vi "시뮬레이터_0720.vi"() -> ()   [LabVIEW 2017]
doc: "This example demonstrates how to continuously acquire buffered voltage measurements using a DAQmx device.\n\nFor instructions on how to connect your signals to the DAQ device, refer to your device documentation."
uses:
  <vilib>/Utility/error.llb/DialogType.ctl
  <vilib>/DAQmx/read.llb/DAQmx Read (Analog 1D Wfm NChan NSamp).vi
  <vilib>/DAQmx/configure/task.llb/DAQmx Configure Logging (TDMS).vi
  <vilib>/DAQmx/miscellaneous.llb/DAQmx Fill In Error Info.vi
  <vilib>/express/express shared/transition.llb/Dynamic To Waveform Array.vi
  <vilib>/express/express arith-compare/Formula/Block/exnFormulaBlock how many pts in the wave.vi
  <vilib>/express/express shared/ex_Modify Signal Name.vi
  <vilib>/express/express shared/transition.llb/Waveform Array To Dynamic.vi
  <vilib>/measure/maspectr.llb/FFT Power Spectrum and PSD for N Chan.vi
  <vilib>/express/express arith-compare/Formula/XNode/ExpressFormulaBlockNode.xnode
  <vilib>/measure/NI_MAPro.lvlib
  SetupDAQ.vi
panel:
  out "불리언 7":bool
  out "불리언 6":bool
  in  "라디오 버튼":T1(radio)
  out "Sensor A Raw 6":dynamicdata(graph)
  in  "Sensor C Channel 2":tag="Dev2/ai0"
  in  "Sensor D Channel 2":tag="Dev2/ai1"
  in  "Terminal config 2":i32(ring)=10083 items=["default"=-1, "RSE"=10083, "NRSE"=10078, "Differential"=10106, "Pseudodifferential"=12529]
  out "A,B Filtering Signal 2":dynamicdata(graph)
  out "55-65(A)":dynamicdata(graph)
  out "55-65(B)":dynamicdata(graph)
  out "10-20(B)":dynamicdata(graph)
  out "10-20(A)":dynamicdata(graph)
  out "불리언 5":bool
  out "불리언 4":bool
  out "불리언 3":bool
  out "불리언 2":bool
  out "A,B Original Signal 2":waveform(dbl)[](graph)
  out "웨이브폼 그래프":dynamicdata(graph)
  out "FFT Power Spectrum 2":dynamicdata(graph)
  out "A,B Filtering Signal":dynamicdata(graph)
  out "Sensor A Raw 5":dynamicdata(graph)
  in  "number of averages":u32=1
  out "Power Spectrum / PSD":cluster{"f0":dbl, "df":dbl, "magnitude":dbl[]}[](graph)
  out "detected amplitudes 2":dbl(graph)=1.1331379876254155
  out "detected frequencies 2":dbl(graph)=60.0
  out "detected frequencies":dbl[](array[numeric])=[60.0, 60.0]
  out "detected amplitudes":dbl[](array[numeric])=[1.1331379876254155, 0.40633237156802526]
  out "Sensor B Raw 2":waveform(dbl)(graph)
  out "Sensor A Raw 2":waveform(dbl)(graph)
  out "B Raw Signal":waveform(dbl)(graph)
  out "A Raw Signal":waveform(dbl)(graph)
  in  "TDMS File Path":path
  in  "Logging Mode":i32(ring)=10231 items=["Off"=10231, "Log and Read"=15842]
  in  "Sensor B Channel":tag="Dev2/ai1"
  in  "Sensor A Channel":tag="Dev2/ai0"
  in  "Terminal config":i32(ring)=10083 items=["default"=-1, "RSE"=10083, "NRSE"=10078, "Differential"=10106, "Pseudodifferential"=12529]
  in  "rate":dbl=5000.0
  out "FFT Power Spectrum":cluster{"f0":dbl, "df":dbl, "magnitude":dbl[]}[](graph)
  in  "Stop":bool
  in  "Number of Samples":i32=100
  # "A신호"
  # "B신호"
  # "Channel Settings"
  # "C신호"
  # "A신호"
  # "D신호"
  # "B신호"
  # "Logging Settings"
  # "A-B Signal Display"
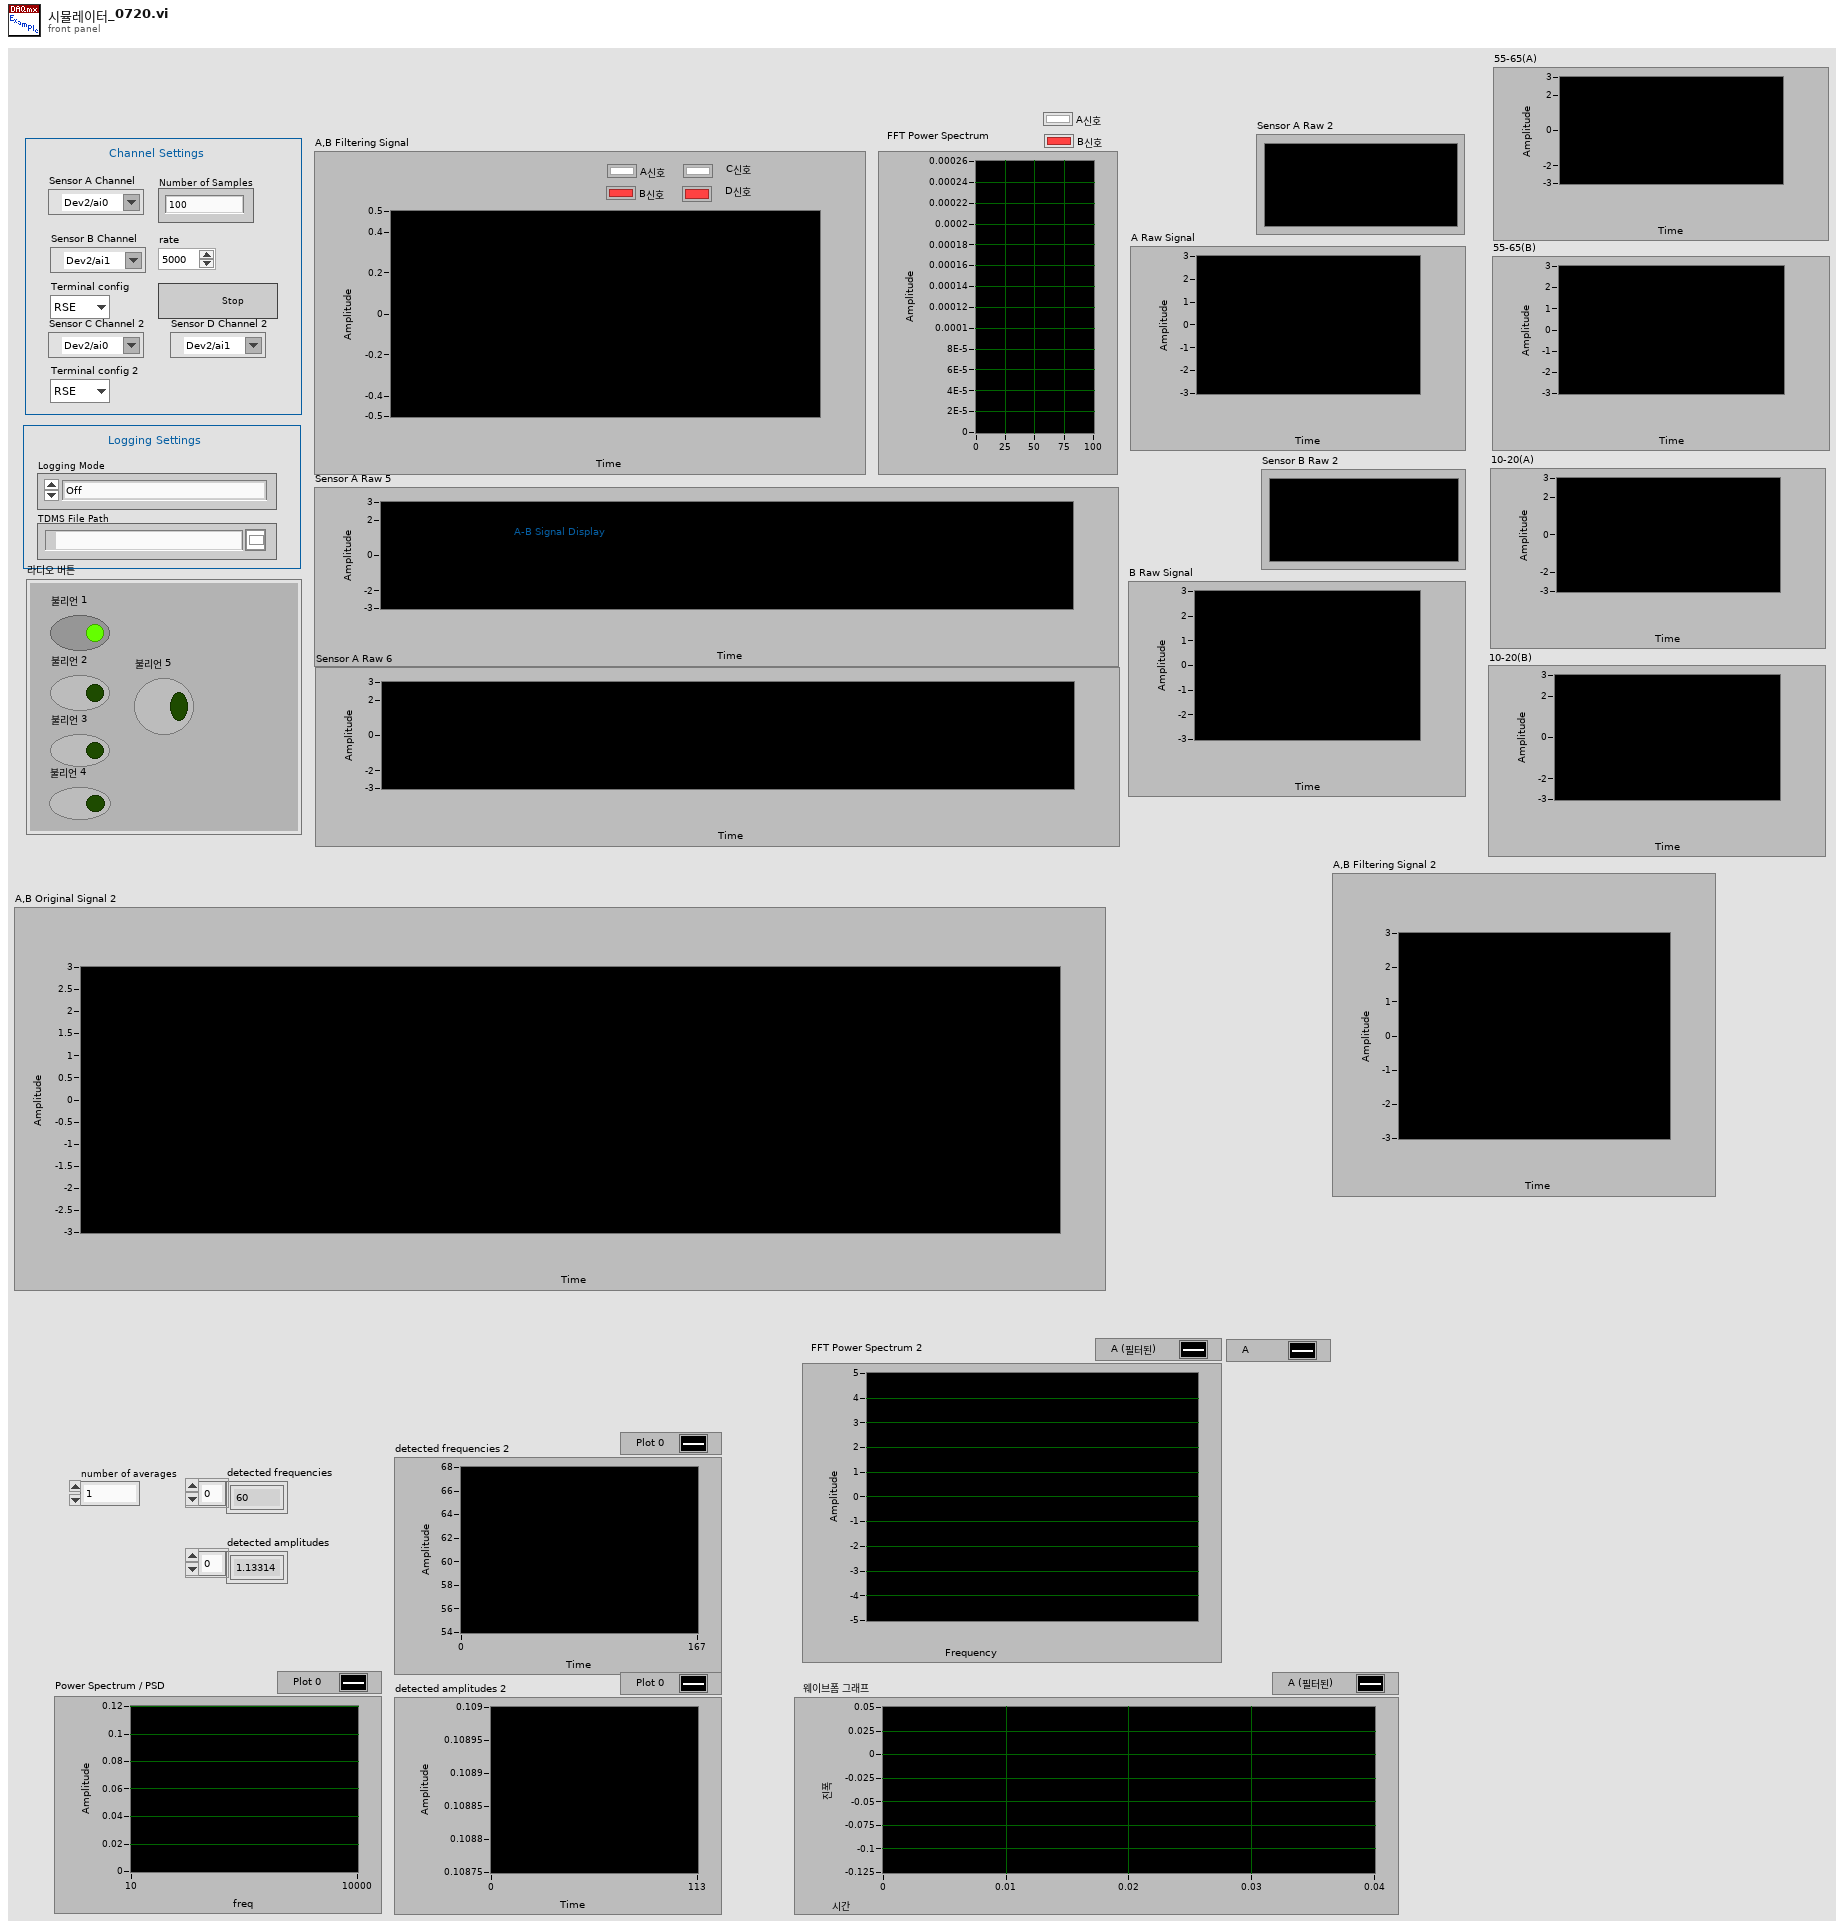
[diagram p1: front panel]
types:
  T1 = enum32{"불리언 1", "불리언 2", "불리언 3", "불리언 4", "불리언 5"}
  T2 = typedef "DialogType.ctl" = u16
  T3 = cluster{"averaging mode":enum16{"No averaging", "Vector averaging", "RMS averaging", "Peak hold"}, "weighting mode":enum16{"Linear", "Exponential"}, "number of averages":u32}
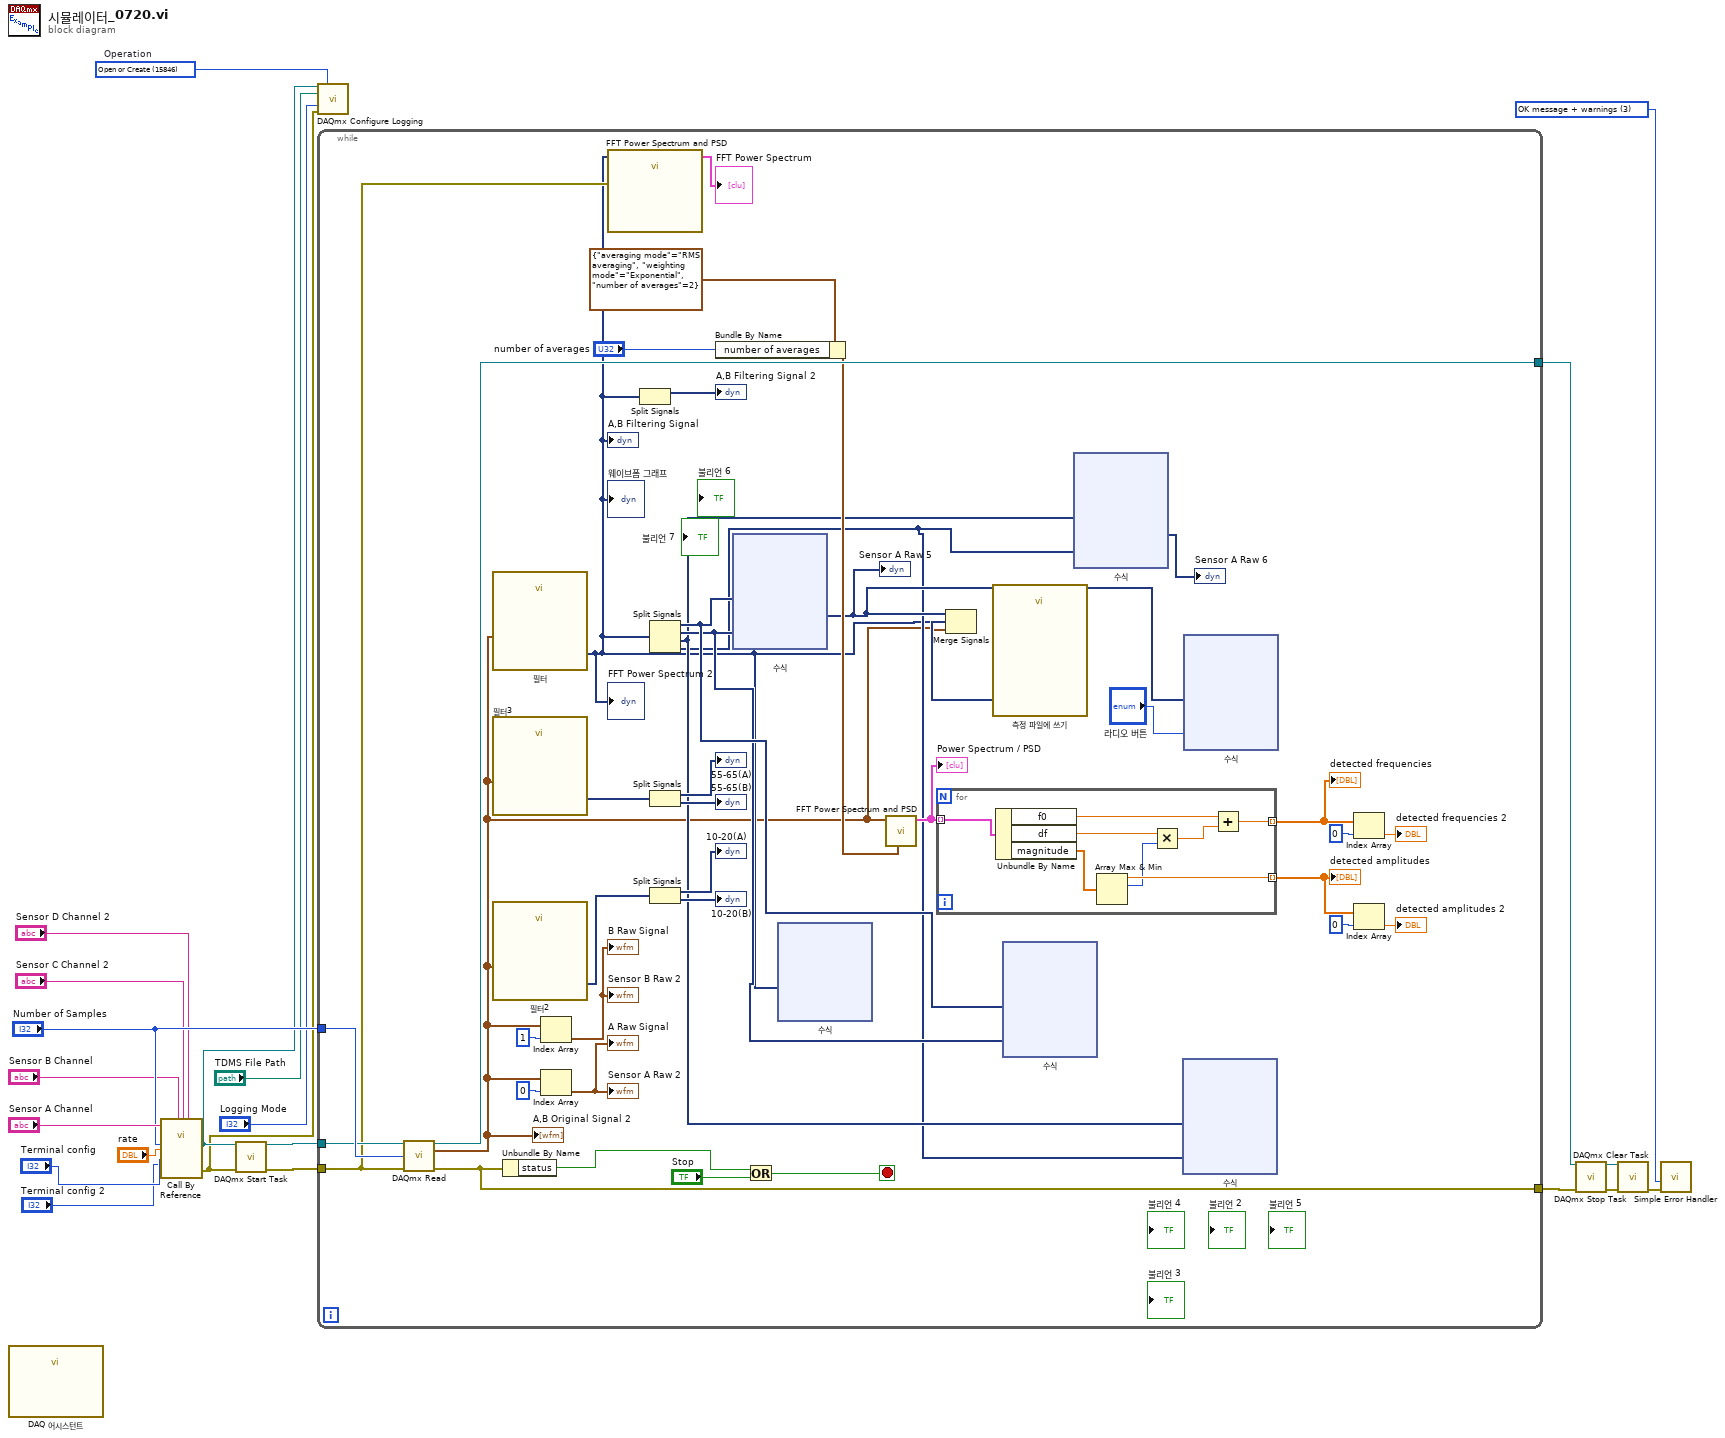
[diagram p0: block diagram]
diagram:
  w10 = 15846 items=["Open"=10437, "Open or Create"=15846, "Create or Replace"=15847, "Create"=15848]  # Operation
  w14 = T2 3 items=["no dialog", "OK message", "continue or stop message", "OK message + warnings", "continue/stop + warnings"] ("type of dialog (OK msg:1)")
  n1 = call "DAQ 어시스턴트"() -> ()  [unwired: 12 in]
  n2 = call-by-ref "?"("number of samples"="Number of Samples", "rate"="rate", "input terminal configuration"="Terminal config", "input terminal configuration 2"="Terminal config 2", "physical channel"="Sensor A Channel", "physical channel 2"="Sensor B Channel", "physical channel 3"="Sensor C Channel 2", "physical channel 4"="Sensor D Channel 2") -> ("task out"=w7:refnum<k21>, "error out"=w6:errorcluster)  [unwired: 12 in, 2 out]
  n3 = call <vilib>:"DAQmx Start Task.vi"("task/channels in"=w7, "error in"=w6) -> ("task out"=w21:refnum<k21>, "error out"=w20:errorcluster)  [unwired: 12 in]
  n4 = call-poly <vilib>:"DAQmx Configure Logging.vi"("task/channels in"=w7, "operation"=w10, "file path"="TDMS File Path", "logging mode"="Logging Mode", "error in"=w6) -> ()  [unwired: 9 in, 2 out]
  n5 = while {
    tunnel: w21 -> [w55]
    tunnel: w20 -> [w54]
    tunnel: [w61] -> w18
    tunnel: [w59] -> w17
    tunnel: "Number of Samples" -> [w56]
    stop <- w57 stop-if-true
    n6 = call-poly <vilib>:"DAQmx Read.vi"("task/channels in"=w55, "number of samples per channel"=w56, "error in"=w54) -> ("task out"=w61:refnum<k21>, "data"=w22:waveform(dbl)[], "error out"=w59:errorcluster)  [unwired: 10 in]
    "A,B Original Signal 2" <- w22
    n7 = call "필터"("Signal"=w22) -> ("Filtered Signal"=w23:dynamicdata)  [unwired: 9 in, 1 out]
    "A,B Filtering Signal" <- w23
    "FFT Power Spectrum 2" <- w23
    "웨이브폼 그래프" <- w23
    n8 = call "필터3"("Signal"=w22) -> ("Filtered Signal"=w32:dynamicdata)  [unwired: 9 in, 1 out]
    n9 = call "필터2"("Signal"=w22) -> ("Filtered Signal"=w37:dynamicdata)  [unwired: 9 in, 1 out]
    n10 = Unbundle By Name(w59) -> ("status"=w58:bool)
    n11 = Index Array(array=w22, index=1) -> (element=→"B Raw Signal" →"Sensor B Raw 2":waveform(dbl))
    n12 = Index Array(array=w22, index=0) -> (element=→"A Raw Signal" →"Sensor A Raw 2":waveform(dbl))
    n13 = call-poly <vilib>:"FFT Power Spectrum and PSD.vi"("error in (no error)"=w54, "time signals"=w23) -> ("Power Spectrum / PSD"=→"FFT Power Spectrum":cluster{"f0":dbl, "df":dbl, "magnitude":dbl[]}[])  [unwired: 6 in, 3 out]
    n14 = Split Signals(w23) -> (→"A,B Filtering Signal 2":dynamicdata)  [unwired: 2 in, 1 out]
    n15 = Split Signals(w23) -> (w27:dynamicdata, w26:dynamicdata, w25:dynamicdata, w24:dynamicdata)  [unwired: 4 in]
    n16 = Split Signals(w32) -> (→"55-65(A)":dynamicdata, →"55-65(B)":dynamicdata)  [unwired: 2 in]
    n17 = Split Signals(w37) -> (→"10-20(A)":dynamicdata, →"10-20(B)":dynamicdata)  [unwired: 2 in]
    n18 = Bundle By Name(cluster=T3 {"averaging mode"=enum."RMS averaging", "weighting mode"=enum."Exponential", "number of averages"=2} ("averaging parameters"), "number of averages"="number of averages") -> (w41:T3)
    n19 = xnode "수식"("X1"=w27, "X2"=w26) -> ("결과"=w29:dynamicdata)  [unwired: 1 in, 1 out]
    "Sensor A Raw 5" <- w29
    n20 = Or(x=w58, y="Stop") -> (x .or. y?=w57:bool)
    n21 = xnode "수식"("X1"=w23) -> ()  [unwired: 1 in, 2 out]
    n22 = call-poly <vilib>:"FFT Power Spectrum and PSD.vi"("averaging parameters"=w41, "time signals"=w22) -> ("Power Spectrum / PSD"=w48:cluster{"f0":dbl, "df":dbl, "magnitude":dbl[]}[])  [unwired: 6 in, 3 out]
    "Power Spectrum / PSD" <- w48
    n23 = for {
      tunnel: w48 -> [w764] mode=indexing
      tunnel: [w762] -> w46 mode=indexing
      tunnel: [w757] -> w43 mode=indexing
      n24 = Unbundle By Name(w764) -> ("f0"=w761:dbl, "df"=w758:dbl, "magnitude"=w763:dbl[])
      n25 = Array Max & Min(array=w763) -> (max value=w762:dbl, max index (indices)=w759:i32)  [unwired: 2 out]
      n26 = Multiply(x=w758, y=w759) -> (x*y=w760:dbl)
      n27 = Add(x=w761, y=w760) -> (x+y=w757:dbl)
    }
    "detected amplitudes" <- w46
    "detected frequencies" <- w43
    n28 = Merge Signals(w29, w23, w22) -> (w38:dynamicdata)
    n29 = call "측정 파일에 쓰기"("Signals"=w38) -> ()  [unwired: 16 in, 3 out]
    n30 = xnode "수식"("X1"=w27, "X2"=w26) -> ()  [unwired: 1 in, 2 out]
    n31 = xnode "수식"("X1"=w25, "X2"=w24) -> ("결과"=→"Sensor A Raw 6":dynamicdata)  [unwired: 1 in, 1 out]
    n32 = xnode "수식"("X1"=w25, "X2"=w24) -> ()  [unwired: 1 in, 2 out]
    n33 = xnode "수식"("X1"=w29, "X2"="라디오 버튼") -> ()  [unwired: 1 in, 2 out]
    n34 = Index Array(array=w43, index=0) -> (element=→"detected frequencies 2":dbl)
    n35 = Index Array(array=w46, index=0) -> (element=→"detected amplitudes 2":dbl)
  }
  n36 = call <vilib>:"DAQmx Stop Task.vi"("task/channels in"=w18, "error in"=w17) -> ("task out"=w15:refnum<k21>, "error out"=w16:errorcluster)  [unwired: 12 in]
  n37 = call <vilib>:"DAQmx Clear Task.vi"("task in"=w15, "error in"=w16) -> ("error out"=w19:errorcluster)  [unwired: 13 in]
  n38 = call <vilib>:"Simple Error Handler.vi"("type of dialog (OK msg:1)"=w14, "error in (no error)"=w19) -> ()  [unwired: 3 in, 5 out]
